vi "Oil Test Sequencer.vi"() -> ()   [LabVIEW 2015]
uses:
  User Interface/Controls/Abort Test.ctl
  User Interface/Controls/Start Test.ctl
  User Interface/Controls/Configuration.ctl
  User Interface/Controls/Manual.ctl
  User Interface/Controls/Quit.ctl
  User Interface/UI Handler/Typedefs/Session Handle.ctl
  User Interface/UI Handler/UI Handler.lvclass
  Tests/Controls/Test Results.ctl
  Tests/Controls/Step Result.ctl
  Tests/Controls/Startup Test.ctl
  Common/Circular Error Log/Typedefs/Session Handle.ctl
  Common/Circular Error Log/Circular Error Log.lvclass
  Tests/Controls/Test Information.ctl
  Tests/Controls/Vacuum Test.ctl
  Tests/Controls/Test Timing.ctl
  Tests/Controls/Vaccum Thresholds.ctl
  Tests/Controls/Helium Test.ctl
  Tests/Controls/Helium Thresholds.ctl
  Tests/Controls/Startup Thresholds.ctl
  User Interface/UI Handler/Typedefs/References.ctl
  Report/Controls/Report Config.ctl
  Common/State Machine/State Machine.lvlib
  Common/Buffers/Snapshot/Snapshot.lvclass
  CAN Communication/Oil/Oil.lvclass
panel:
  in  "Quit":T1
  in  "Manual":T2
  in  "Configuration":T3
  in  "Start Test":T4
  in  "Abort Test":T5
  in  "Configuration Files Path":path=path "C:/TMxFlexTests/OC Assembly Tests/Configuration/ProductionTestConfig.xml"
  in  "User":string
  in  "Serial Number":string="OCxxxxxx"
  in  "Test":string
  out "Time Remaining (s)":dbl
  out "Current Step":dbl
  out "Leak Rate":dbl caption="Leak Rate (PSI/s)" format="%.3f"
  out "NI-DAQ":dbl caption="Test Pressure (PSI)" format="%.3f"
  out "exit":bool
  in  "Display":string
  in  "Test Sequence":i32(listbox)=-2
  in  "Message Log":string
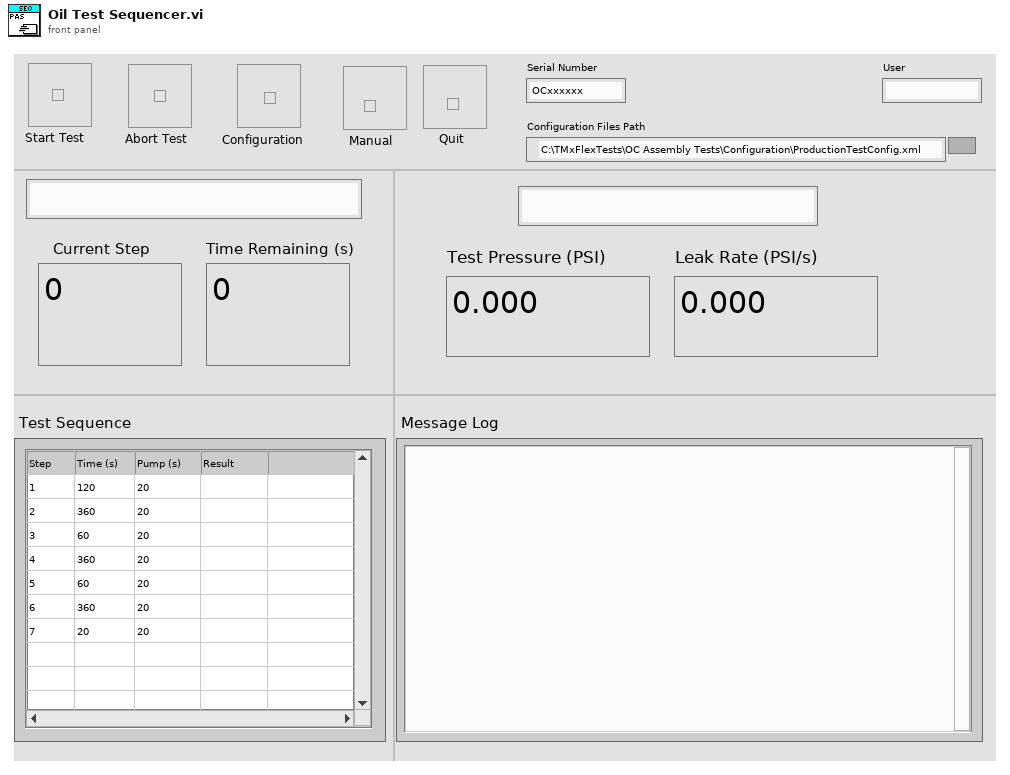
[diagram p1: front panel]
types:
  T1 = typedef "Quit.ctl" = bool
  T2 = typedef "Manual.ctl" = bool
  T3 = typedef "Configuration.ctl" = bool
  T4 = typedef "Start Test.ctl" = bool
  T5 = typedef "Abort Test.ctl" = bool
  T6 = enum8{"Enabled", "Disabled", "Disabled and Grayed Out"}
  T7 = typedef "UI Handler.lvclass/Session Handle.ctl" = refnum<data-value>
  T8 = typedef "Test Results.ctl" = cluster{"Vacuum Test":T9[], "Helium Test":T9[], "Aborted?":bool, "Reason":string, "Abort Time":timestamp, "Test Start":timestamp, "Test End":timestamp, "Startup Test":T10}
  T9 = typedef "Step Result.ctl" = cluster{"Functional Pressure":dbl, "Leak Pressure":dbl, "Func Pass?":bool, "Leak Pass?":bool, "Step Start":timestamp, "Step End":timestamp}
  T10 = typedef "Startup Test.ctl" = cluster{"MIO":dbl, "Temperature":dbl, "MIO Pass?":bool, "Temperature Pass?":bool, "Startup Test Pass?":bool, "Startup Test Start":timestamp, "Startup Test End":timestamp, "Pressure Pass?":bool, "Pressure":dbl}
  T11 = typedef "Circular Error Log.lvclass/Session Handle.ctl" = refnum<data-value>
  T12 = typedef "Test Information.ctl" = cluster{"Vacuum Test":T13, "Helium Test":T16, "Startup Thresholds":T18}
  T13 = typedef "Vacuum Test.ctl" = cluster{"Vacuum Timings":T14[], "Vacuum Thresholds":T15[], "Leak Reasons":string[], "Func Reasons":string[], "FuncSpecEqual":string[], "LeakSpecEqual":string[]}
  T14 = typedef "Test Timing.ctl" = cluster{"Step Wait":dbl, "Pump Wait":dbl}
  T15 = typedef "Vaccum Thresholds.ctl" = cluster{"Func Max Pressure":dbl, "Func Min Pressure":dbl, "Leak Max Pressure":dbl, "Leak Min Pressure":dbl}
  T16 = typedef "Helium Test.ctl" = cluster{"Helium Timings":T14[], "Helium Thresholds":T17[], "Failure Reasons":string[], "LeakSpecEqual":string[]}
  T17 = typedef "Helium Thresholds.ctl" = cluster{"Leak Max Pressure":dbl, "Leak Min Pressure":dbl}
  T18 = typedef "Startup Thresholds.ctl" = cluster{"MIO Max":dbl, "MIO Min":dbl, "Temp Max":dbl, "Temp Min":dbl, "Pressure Max":dbl, "Pressure Min":dbl}
  T19 = cluster{"State":refnum<queue>, "UI Handler":T7, "Serial Number":string, "Test Type":string, "Test Results":T8, "Error":T11, "Operator":string, "config path":path, "Test Configuration":T12}
  T20 = typedef "UI Handler.lvclass/References.ctl" = cluster{"Step":refnum<vi>, "Time":refnum<vi>, "Sequencer":refnum<vi>, "Log":refnum<vi>}
  T21 = cluster{"Serial Number Out":string, "Operator":string}
  T22 = typedef "Report Config.ctl" = cluster{"Serial Number":string, "Test Results":T8, "Operator":string, "Config Filepath":path, "Test Information":T12}
  T23 = typedef "Oil.lvclass/Session Handle.ctl" = refnum<data-value>
  T24 = typedef "Snapshot.lvclass/Session Handle.ctl" = refnum<data-value>
  T25 = typedef "User Configuration.ctl" = cluster{"Password":string, "cDAQ Name":string, "CAN Interface":string}
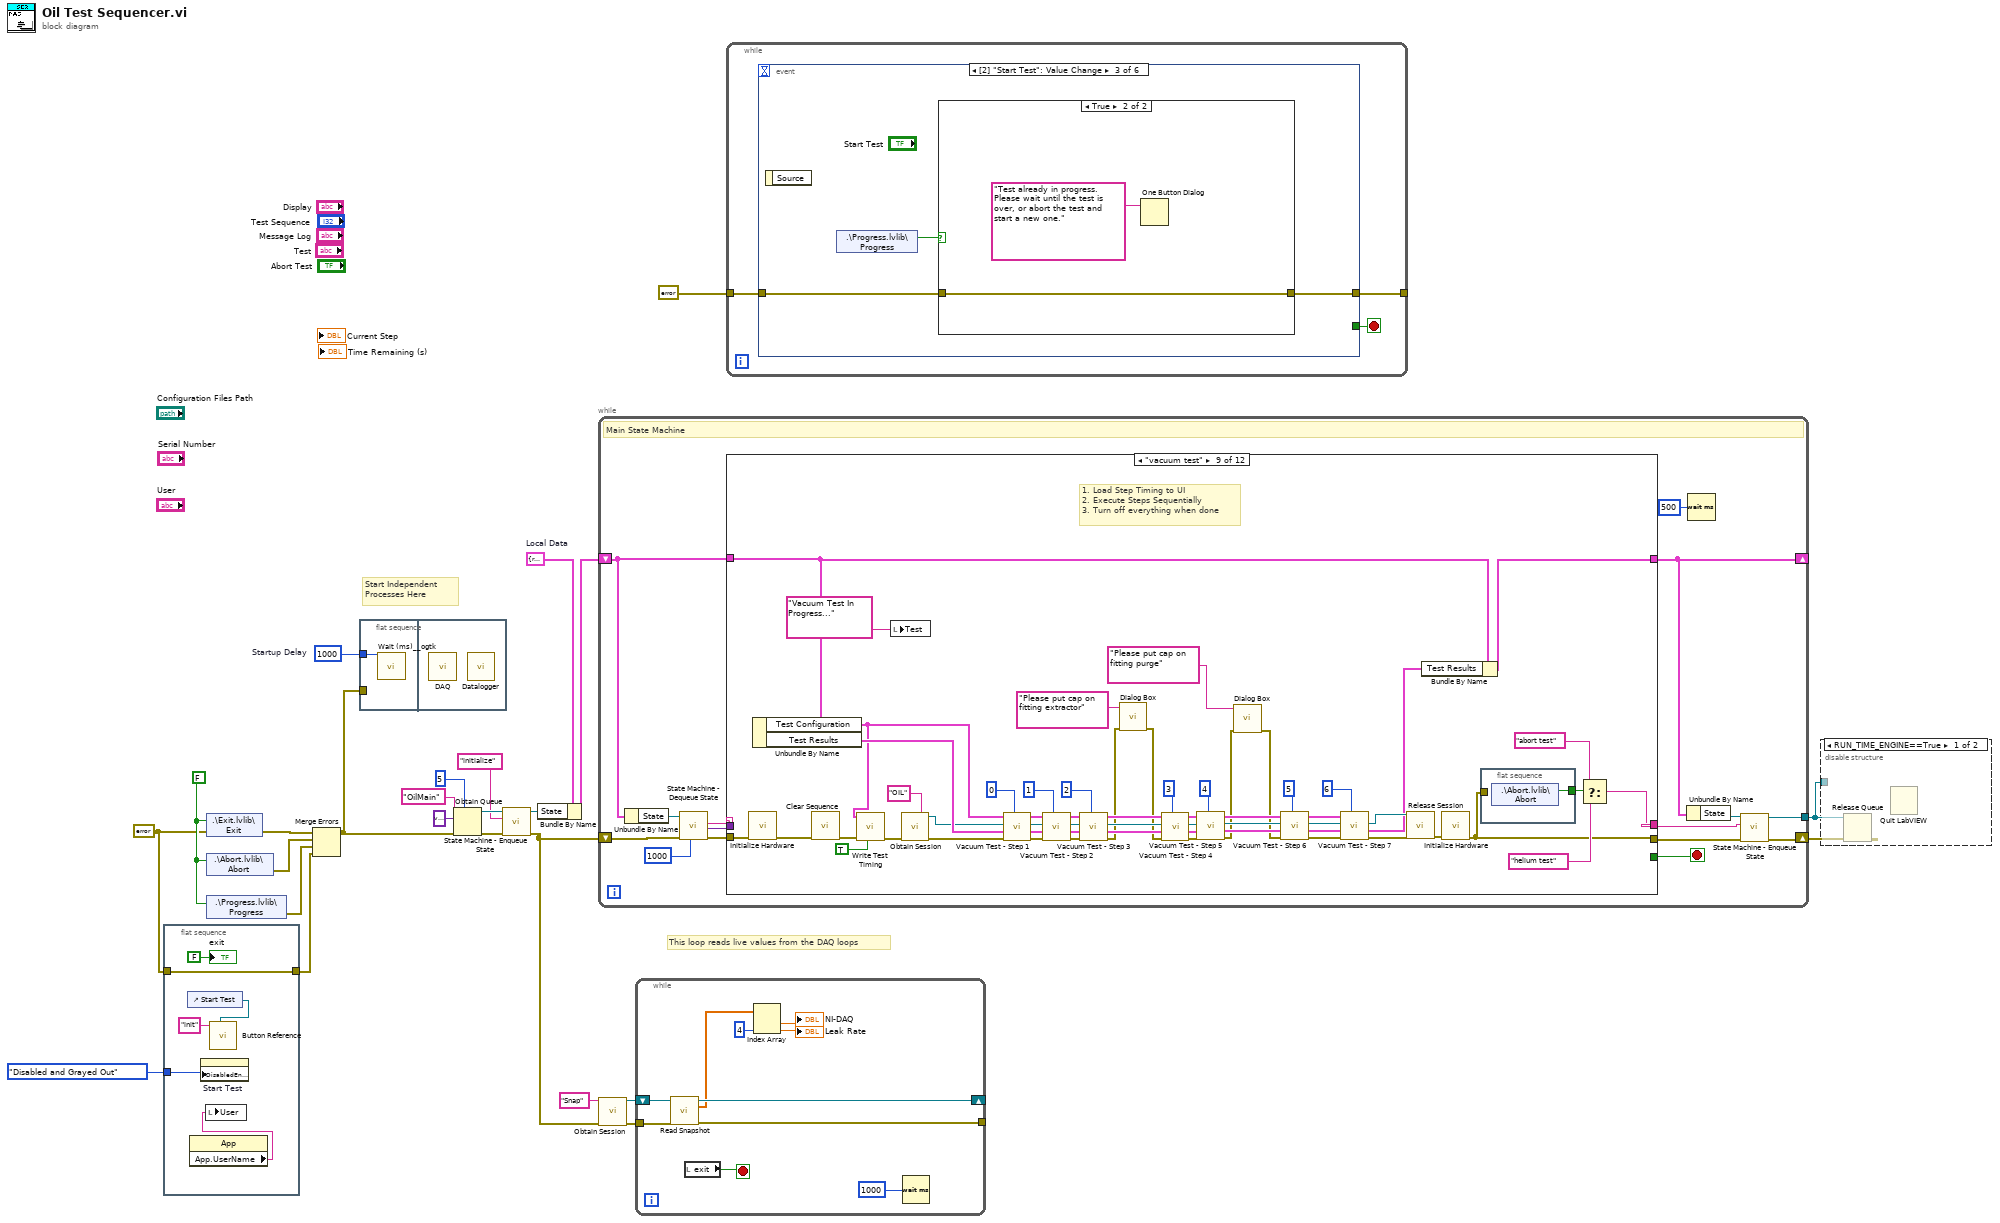
[diagram p0: block diagram]
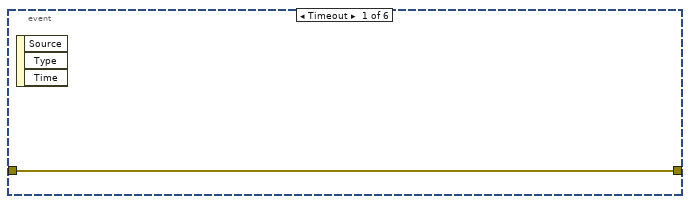
[diagram p3: hidden frame]
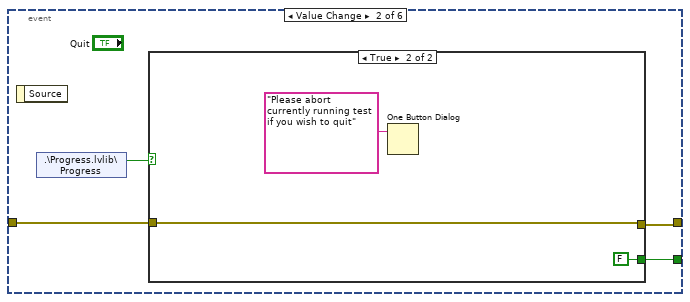
[diagram p4: hidden frame]
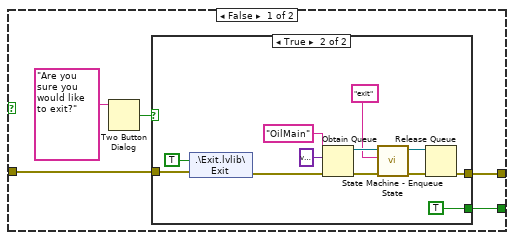
[diagram p5: hidden frame]
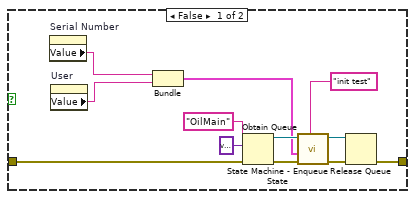
[diagram p7: hidden frame]
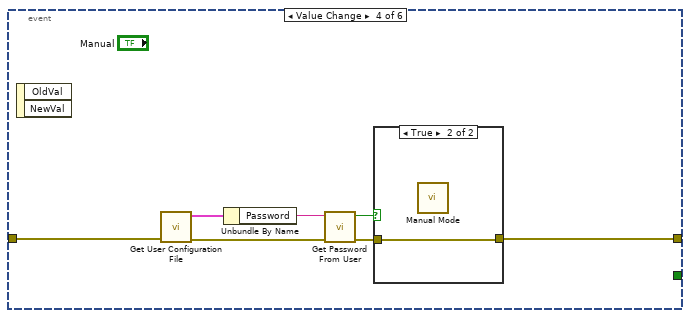
[diagram p8: hidden frame]
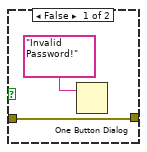
[diagram p9: hidden frame]
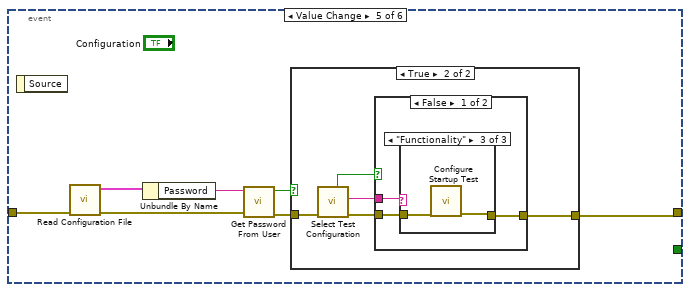
[diagram p10: hidden frame]
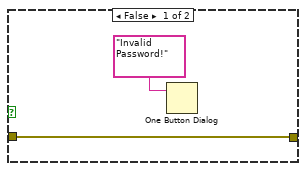
[diagram p11: hidden frame]
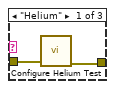
[diagram p12: hidden frame]
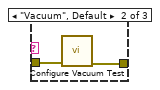
[diagram p13: hidden frame]
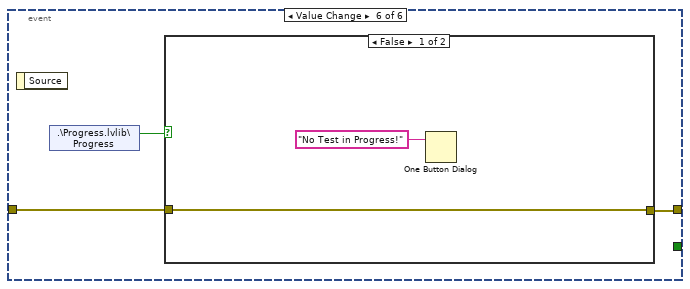
[diagram p15: hidden frame]
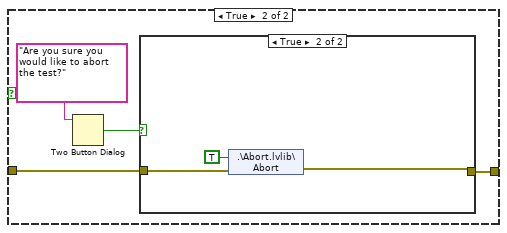
[diagram p16: hidden frame]
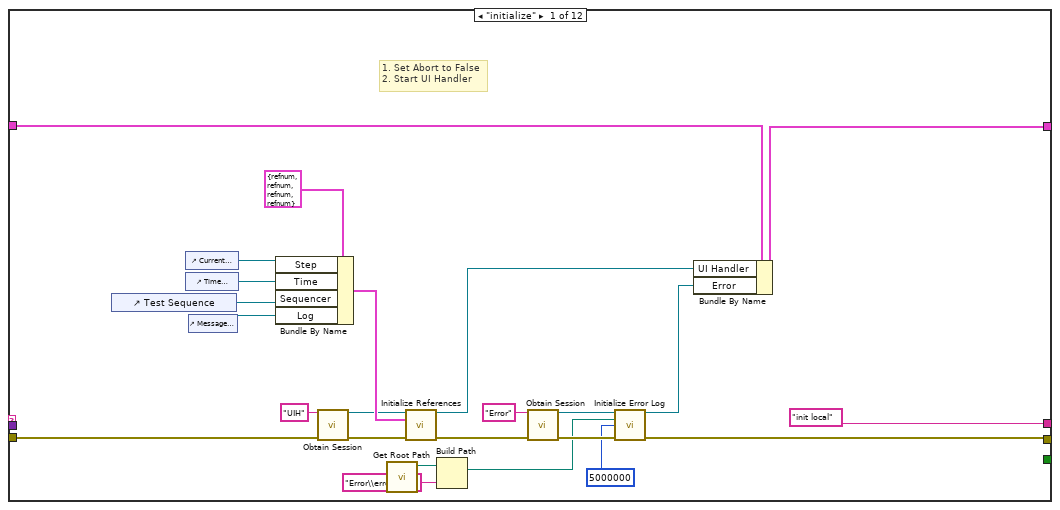
[diagram p18: hidden frame]
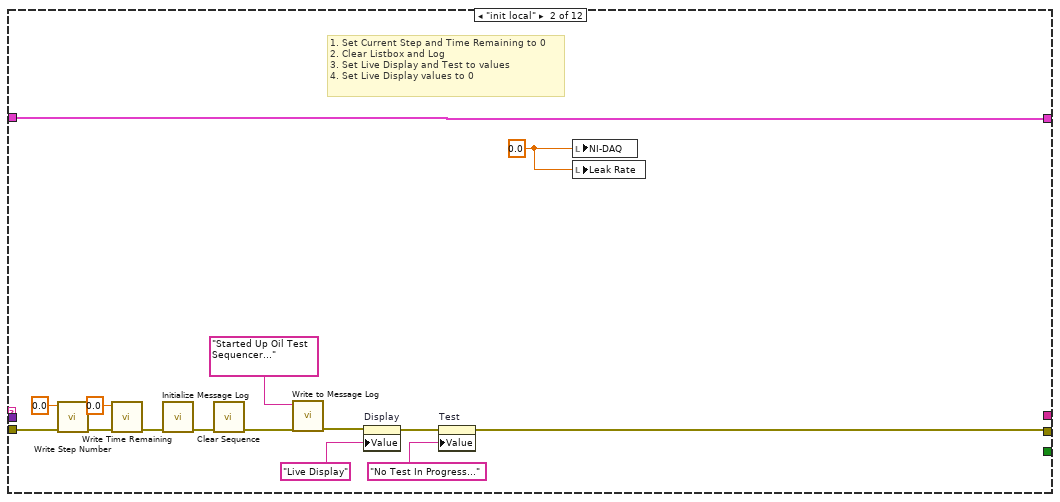
[diagram p19: hidden frame]
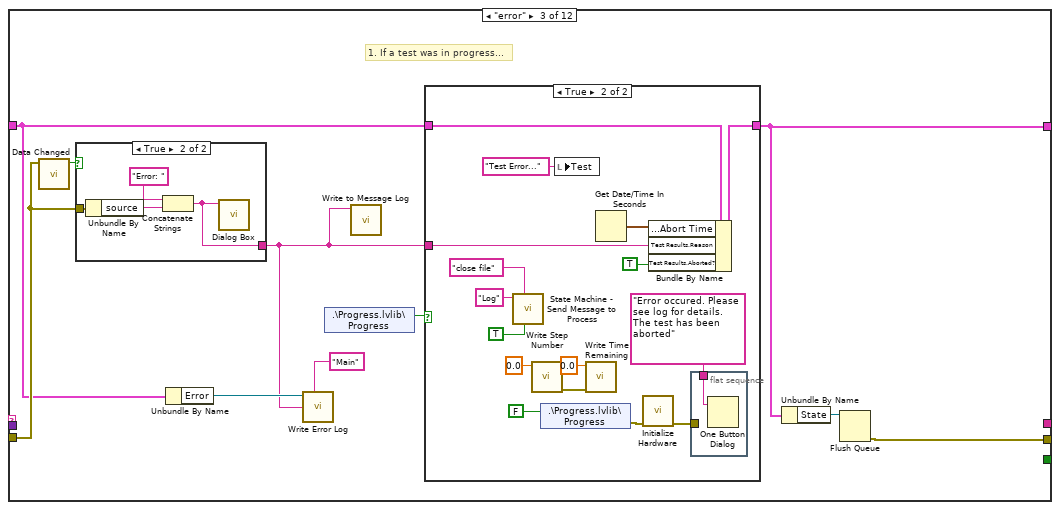
[diagram p20: hidden frame]
diagram:
  w10 = FALSE ("Exit")
  w16 = u32 1000  # Startup Delay
  w4 = errorcluster {"status"=FALSE, "code"=0, "source"=""} ("error in (no error)")
  w19 = T19 {"State"=refnum, "UI Handler"=refnum, "Serial Number"="", "Test Type"="", "Test Results"={"Vacuum Test"=[], "Helium Test"=[], "Aborted?"=FALSE, "Reason"="", "Abort Time"=timestamp(0 s since 1904-01-01), "Test Start"=timestamp(0 s since 1904-01-01), "Test End"=timestamp(0 s since 1904-01-01), "Startup Test"={"MIO"=0.0, "Temperature"=0.0, "MIO Pass?"=FALSE, "Temperature Pass?"=FALSE, "Startup Test Pass?"=FALSE, "Startup Test Start"=timestamp(0 s since 1904-01-01), "Startup Test End"=timestamp(0 s since 1904-01-01), "Pressure Pass?"=FALSE, "Pressure"=0.0}}, "Error"=refnum, "Operator"="", "config path"=path "", "Test Configuration"={"Vacuum Test"={"Vacuum Timings"=[], "Vacuum Thresholds"=[], "Leak Reasons"=[], "Func Reasons"=[], "FuncSpecEqual"=[], "LeakSpecEqual"=[]}, "Helium Test"={"Helium Timings"=[], "Helium Thresholds"=[], "Failure Reasons"=[], "LeakSpecEqual"=[]}, "Startup Thresholds"={"MIO Max"=0.0, "MIO Min"=0.0, "Temp Max"=0.0, "Temp Min"=0.0, "Pressure Max"=0.0, "Pressure Min"=0.0}}}  # Local Data
  # "This loop reads live values from the DAQ loops"
  # "Start Independent\nProcesses Here"
  n1 = flat-sequence {
    tunnel: w4 -> [w30]
    tunnel: [w30] -> w3
    tunnel: T6."Disabled and Grayed Out" ("Disabled") -> [w28]
    frame #0 {
      n2 = control-ref of="Start Test"() -> (w29:refnum<vi>)
      n3 = property class="App"() -> ("App.UserName"=w26:string)  [unwired: 2 in, 2 out]
      n4 = property on="Start Test" class="Bool"("DisabledEnum"=w28) -> ()  [unwired: 2 in, 2 out]
      n5 = local write "User"(w26) -> ()
      n6 = call "Button Reference.vi"("Ref In"=w29, "Command"="init") -> ()  [unwired: 9 in, 1 out]
      "exit" <- FALSE ("exit")
    }
  }
  n7 = shared-variable ".\\Exit.lvlib\\Exit"(w10, error in=w4) -> (error out=w14:errorcluster)
  n8 = shared-variable ".\\Abort.lvlib\\Abort"(w10) -> (error out=w15:errorcluster)  [unwired: 1 in]
  n9 = shared-variable ".\\Progress.lvlib\\Progress"(w10) -> (error out=w9:errorcluster)  [unwired: 1 in]
  n10 = Merge Errors(w14, w15, w9, w3) -> (w13:errorcluster)
  n11 = flat-sequence {
    tunnel: w13 -> [_]
    tunnel: w16 -> [w32]
    frame #0 {
      n12 = call <userlib>:"Wait (ms)__ogtk.vi"("milliseconds to wait"=w32) -> ()  [unwired: 9 in, 2 out]
    }
    frame #1 {
      n13 = call "DAQ.vi"() -> ()  [unwired: 12 in]
      n14 = call "Datalogger.vi"() -> ()  [unwired: 12 in]
    }
  }
  n15 = Obtain Queue(max queue size (-1, unlimited)=5, name (unnamed)="OilMain", element data type=variant, error in (no error)=w13) -> (queue out=w21:refnum<queue>, error out=w22:errorcluster)  [unwired: 1 in, 1 out]
  n16 = call "State Machine - Enqueue State.vi"("error in (no error)"=w22, "State"="initialize", "Queue In"=w21) -> ("error out"=w7:errorcluster, "Queue Out"=w18:refnum<queue>)  [unwired: 7 in]
  n17 = Bundle By Name(cluster=w19, "State"=w18) -> (w17:T19)
  n18 = while "Main State Machine" {
    shift-right: [w44] -> w11
    shift-left: w7 -> [w47]
    shift-right: [w35] -> _
    shift-left: w17 -> [w38]
    tunnel: [w33] -> w2
    stop <- w40 stop-if-true
    # "Main State Machine"
    n19 = Unbundle By Name(w38) -> ("State"=w37:refnum<queue>)
    n20 = call "State Machine - Dequeue State.vi"("Timeout"=1000, "error in (no error)"=w47, "Queue In"=w37) -> ("error out"=w46:errorcluster, "Data"=w34:variant, "State"=w45:string)  [unwired: 4 in, 2 out]
    n21 = case shown="\"vacuum test\"" w45 {
      tunnel: w46 -> [w61 w85 w90 w124 w126 w133 w175 w185 w236 w274 w314 w326]
      tunnel: [w52 w73 w96 w124 w126 w134 w153 w176 w235 w277 w290 w324] -> w43
      tunnel: ["init local" ("State") _ _ _ _ _ w169 "vacuum test" ("Next Test") w237 w278 _ _] -> w42
      tunnel: [_ _ _ _ _ TRUE _ _ _ _ _ _] -> w40
      tunnel: w38 -> [w60 w86 w89 w123 w125 w140 w172 w182 w242 w283 w310 w323]
      tunnel: [w59 w86 w94 w123 w125 w140 w173 w184 w241 w282 w310 w323] -> w35
      tunnel: w34 -> [_ _ _ _ _ _ w174 _ _ _ _ _]
      frame "initialize" {
        # "1. Set Abort to False\n2. Start UI Handler"
        n22 = control-ref of="Test Sequence"() -> (w64:refnum<vi>)
        n23 = control-ref of="Current Step"() -> (w62:refnum<vi>)
        n24 = control-ref of="Time Remaining (s)"() -> (w63:refnum<vi>)
        n25 = control-ref of="Message Log"() -> (w65:refnum<vi>)
        n26 = Bundle By Name(cluster=T20 {"Step"=refnum, "Time"=refnum, "Sequencer"=refnum, "Log"=refnum} ("References"), "Step"=w62, "Time"=w63, "Sequencer"=w64, "Log"=w65) -> (w70:T20)
        n27 = call "Obtain Session.vi"("Session  Name ()"="UIH", "error in (no error)"=w61) -> ("Session Handle"=w68:T7, "error out"=w69:errorcluster)  [unwired: 12 in]
        n28 = call "Get Root Path.vi"() -> ("Root Path"=w50:path)  [unwired: 11 in]
        n29 = call "Initialize References.vi"("Session Handle in"=w68, "References"=w70, "error in (no error)"=w69) -> ("Session Handle out"=w58:T7, "error out"=w57:errorcluster)  [unwired: 11 in]
        n30 = Build Path(base path=w50, name or relative path="Error\\error.txt") -> (appended path=w48:path)
        n31 = call "Obtain Session.vi"("Session  Name ()"="Error", "error in (no error)"=w57) -> ("Session Handle"=w54:T11, "error out"=w55:errorcluster)  [unwired: 12 in]
        n32 = call "Initialize Error Log.vi"("Session Handle in"=w54, "Error Path"=w48, "Max File Size"=i64 5000000, "error in (no error)"=w55) -> ("Session Handle out"=w51:T11, "error out"=w52:errorcluster)  [unwired: 10 in]
        n33 = Bundle By Name(cluster=w60, "UI Handler"=w58, "Error"=w51) -> (w59:T19)
      }
      frame "init local" {
        w72 = 0.0 ("Test Pressure (PSI)")
        # "1. Set Current Step and Time Remaining to 0\n2. Clear Listbox and Log\n3. Set Live Display and Test to values \n4. Set Live Display values to 0"
        n34 = call "Write Step Number.vi"("error in (no error)"=w85, "Value"=0.0) -> ("error out"=w83:errorcluster)  [unwired: 9 in]
        n35 = call "Write Time Remaining.vi"("error in (no error)"=w83, "Value"=0.0) -> ("error out"=w81:errorcluster)  [unwired: 9 in]
        n36 = call "Initialize Message Log.vi"("error in (no error)"=w81) -> ("error out"=w80:errorcluster)  [unwired: 10 in]
        n37 = call "Clear Sequence.vi"("error in (no error)"=w80) -> ("error out"=w79:errorcluster)  [unwired: 10 in]
        n38 = call "Write to Message Log.vi"("error in (no error)"=w79, "Message"="Started Up Oil Test Sequencer...") -> ("error out"=w77:errorcluster)  [unwired: 9 in]
        n39 = property on="Display" class="Str"(error in=w77, "Value"="Live Display" ("Display")) -> (error out=w75:errorcluster)  [unwired: 1 in, 1 out]
        n40 = property on="Test" class="Str"(error in=w75, "Value"="No Test In Progress..." ("Test")) -> (error out=w73:errorcluster)  [unwired: 1 in, 1 out]
        n41 = local write "NI-DAQ"(w72) -> ()
        n42 = local write "Leak Rate"(w72) -> ()
      }
      frame "error" {
        # "1. If a test was in progress..."
        n43 = call "Data Changed.vi"("Data"=w90) -> ("Changed?"=w92:bool)  [unwired: 10 in]
        n44 = case shown="True" w92 {
          tunnel: [w97 w101] -> w87
          tunnel: w90 -> [w98 w102]
          frame False {
            n45 = Unbundle By Name(w98) -> ("source"=w99:string)
            n46 = Concatenate Strings("Error: " ("string"), w99) -> (w97:string)
          }
          frame True {
            n47 = Unbundle By Name(w102) -> ("source"=w103:string)
            n48 = Concatenate Strings("Error: " ("string"), w103) -> (w101:string)
            n49 = call "Dialog Box.vi"("Serial Number"=w101) -> ()  [unwired: 10 in, 1 out]
          }
        }
        n50 = Unbundle By Name(w89) -> ("Error"=w88:T11)
        n51 = call "Write Error Log.vi"("Session Handle in"=w88, "Process Name"="Main", "Data"=w87) -> ()  [unwired: 11 in, 2 out]
        n52 = shared-variable ".\\Progress.lvlib\\Progress"() -> (w93:bool)  [unwired: 1 in, 1 out]
        n53 = call "Write to Message Log.vi"("Message"=w87) -> ()  [unwired: 10 in, 1 out]
        n54 = case shown="True" w93 {
          tunnel: w89 -> [w105 w120]
          tunnel: [w105 w119] -> w94
          tunnel: w87 -> [_ w117]
          frame False {
          }
          frame True {
            n55 = call "State Machine - Send Message to Process.vi"("Front?"=TRUE, "State"="close file", "Process Name"="Log") -> ()  [unwired: 8 in, 1 out]
            n56 = call "Write Step Number.vi"("Value"=0.0) -> ("error out"=w110:errorcluster)  [unwired: 10 in]
            n57 = shared-variable ".\\Progress.lvlib\\Progress"(FALSE ("Progress")) -> (error out=w115:errorcluster)  [unwired: 1 in]
            n58 = local write "Test"("Test Error..." ("Test")) -> ()
            n59 = call "Write Time Remaining.vi"("error in (no error)"=w110, "Value"=0.0) -> ()  [unwired: 9 in, 1 out]
            n60 = Get Date/Time In Seconds() -> (seconds since 1Jan1904=w118:timestamp)
            n61 = call "Initialize Hardware.vi"("error in"=w115) -> ("error out"=w114:errorcluster)  [unwired: 10 in]
            n62 = Bundle By Name(cluster=w120, "Test Results.Abort Time"=w118, "Test Results.Reason"=w117, "Test Results.Aborted?"=TRUE) -> (w119:T19)
            n63 = flat-sequence {
              tunnel: w114 -> [_]
              tunnel: "Error occured. Please see log for details. The test has been aborted" -> [w122]
              frame #0 {
                n64 = One Button Dialog(message=w122) -> ()  [unwired: 1 in, 1 out]
              }
            }
          }
        }
        n65 = Unbundle By Name(w94) -> ("State"=w95:refnum<queue>)
        n66 = Flush Queue(queue=w95) -> (error out=w96:errorcluster)  [unwired: 1 in, 2 out]
      }
      frame Default {
      }
      frame "idle" {
      }
      frame "exit" {
        # "1. Clean up all references\n2. Exit commands to Datalogger"
        n67 = Unbundle By Name(w140) -> ("UI Handler"=w139:T7)
        n68 = call "Write to Message Log.vi"("error in (no error)"=w133, "Message"="Initializing Hardware before exit") -> ("error out"=w132:errorcluster)  [unwired: 9 in]
        n69 = call "Initialize Hardware.vi"("error in"=w132) -> ("error out"=w130:errorcluster)  [unwired: 10 in]
        n70 = call "Release Session.vi"("Session Handle"=w139, "error in (no error)"=w130) -> ()  [unwired: 13 in, 1 out]
        n71 = local write "exit"(TRUE ("exit")) -> ()
        n72 = call "State Machine - Send Message to Process.vi"("Front?"=TRUE, "State"="exit", "Process Name"="DAQ") -> ("error out"=w134:errorcluster)  [unwired: 8 in]
        n73 = call "State Machine - Send Message to Process.vi"("Front?"=TRUE, "State"="exit", "Process Name"="Log") -> ()  [unwired: 8 in, 1 out]
      }
      frame "init test" {
        # "Read test config"
        # "1. Initialize all Hardware\n2. Store Serial Number\n3. Send start command to logger\n4.. Proceed to Test"
        n74 = Variant To Data(error in=w175, type=T21 {"Serial Number Out"="", "Operator"=""} ("cluster"), Variant=w174) -> (data=w168:T21, error out=w145:errorcluster)
        n75 = property on="Configuration Files Path" class="Path"() -> ("Value"=w142:path)  [unwired: 2 in, 2 out]
        n76 = call "Read Test Information From File.vi"("error in"=w145, "file (use dialog)"=w142) -> ("error out"=w144:errorcluster, "Test Information"=w143:T12)  [unwired: 8 in]
        n77 = call "Obtain Session.vi"("Session  Name ()"="OIL", "error in (no error)"=w144) -> ("Session Handle"=w162:T23, "error out"=w163:errorcluster)  [unwired: 12 in]
        n78 = call "Get Device Status.vi"("Session Handle in"=w162, "error in (no error)"=w163) -> ("Session Handle out"=w159:T23, "error out"=w161:errorcluster)  [unwired: 11 in, 1 out]
        n79 = Unbundle By Name(w168) -> ("Operator"=w165:string, "Serial Number Out"=w147:string)
        n80 = call "Write to Message Log.vi"("error in (no error)"=w161, "Message"="Initializing Hardware...") -> ("error out"=w158:errorcluster)  [unwired: 9 in]
        n81 = call "Initialize Hardware.vi"("error in"=w158) -> ("error out"=w148:errorcluster)  [unwired: 10 in]
        n82 = call "WriteVerify Mfg Serial Number.vi"("error in"=w148, "Serial Number"=w147) -> ("error out"=w146:errorcluster)  [unwired: 9 in]
        n83 = Bundle("Serial Number Out"=w147) -> (w149:cluster{"Serial Number Out":string})  [unwired: 1 in]
        n84 = call "State Machine - Send Message to Process.vi"("Data"=w149, "Front?"=TRUE, "State"="create path", "Process Name"="Log") -> ()  [unwired: 7 in, 1 out]
        n85 = call "Release Session.vi"("Session Handle"=w159, "error in (no error)"=w146) -> ("error out"=w156:errorcluster)  [unwired: 13 in]
        n86 = call "Dialog Box.vi"("error in (no error)"=w156, "Serial Number"="Please ensure that there is a cap on the CHV 1 PSI Fitting. Extractor and purge fittings should not be capped.") -> ("error out"=w154:errorcluster)  [unwired: 9 in]
        n87 = Bundle By Name(cluster=w172, "Test Results"=T8 {"Vacuum Test"=[], "Helium Test"=[], "Aborted?"=FALSE, "Reason"="", "Abort Time"=timestamp(0 s since 1904-01-01), "Test Start"=timestamp(0 s since 1904-01-01), "Test End"=timestamp(0 s since 1904-01-01), "Startup Test"={"MIO"=0.0, "Temperature"=0.0, "MIO Pass?"=FALSE, "Temperature Pass?"=FALSE, "Startup Test Pass?"=FALSE, "Startup Test Start"=timestamp(0 s since 1904-01-01), "Startup Test End"=timestamp(0 s since 1904-01-01), "Pressure Pass?"=FALSE, "Pressure"=0.0}}, "Operator"=w165, "Serial Number"=w147, "config path"=w142, "Test Configuration"=w143) -> (w173:T19)
        n88 = call "Clear Sequence.vi"("error in (no error)"=w154) -> ("error out"=w153:errorcluster)  [unwired: 10 in]
        n89 = Select(t="startup test" ("Error String"), s=TRUE ("Progress"), f="idle" ("Error String")) -> (s? t:f=w169:string)
      }
      frame "startup test" {
        # "1. Oil Pump Test\n2. MIO , Temp, Pressure readings"
        n90 = shared-variable ".\\Progress.lvlib\\Progress"(TRUE ("Progress"), error in=w185) -> (error out=w180:errorcluster)
        n91 = Unbundle By Name(w182) -> ("Test Configuration"=w181:T12, "Test Results"=w179:T8)
        n92 = local write "Test"("Startup Test in Progress..." ("Test")) -> ()
        n93 = call "Startup Test.vi"("error in"=w180, "Test Results In"=w179, "Test Configuration In"=w181) -> ("error out"=w176:errorcluster, "Test Results Out"=w178:T8)  [unwired: 6 in, 1 out]
        n94 = Bundle By Name(cluster=w182, "Test Results"=w178) -> (w184:T19)
      }
      frame "vacuum test" {
        # "1. Load Step Timing to UI\n2. Execute Steps Sequentially\n3. Turn off everything when done"
        n95 = call "Initialize Hardware.vi"("error in"=w236) -> ("error out"=w233:errorcluster)  [unwired: 10 in]
        n96 = Unbundle By Name(w242) -> ("Test Configuration"=w207:T12, "Test Results"=w234:T8)
        n97 = call "Clear Sequence.vi"("error in (no error)"=w233) -> ("error out"=w232:errorcluster)  [unwired: 10 in]
        n98 = call "Write Test Timing.vi"("Vacuum?"=TRUE, "error in (no error)"=w232, "Test Configuration"=w207) -> ("error out"=w228:errorcluster)  [unwired: 8 in]
        n99 = local write "Test"("Vacuum Test In Progress..." ("Test")) -> ()
        n100 = call "Obtain Session.vi"("Session  Name ()"="OIL", "error in (no error)"=w228) -> ("Session Handle"=w195:T23, "error out"=w196:errorcluster)  [unwired: 12 in]
        n101 = call "Vacuum Test - Step 1.vi"("Step"=0, "error in"=w196, "Test Results"=w234, "Oil In"=w195, "Test Configuration"=w207) -> ("error out"=w226:errorcluster, "Test Results Out"=w225:T8, "Oil Out"=w224:T23, "Test Configuration Out"=w223:T12)  [unwired: 3 in]
        n102 = call "Vacuum Test - Step 2.vi"("Step"=1, "error in"=w226, "Test Results"=w225, "Oil In"=w224, "Test Configuration"=w223) -> ("error out"=w221:errorcluster, "Test Results Out"=w220:T8, "Oil Out"=w219:T23, "Test Configuration Out"=w218:T12)  [unwired: 3 in]
        n103 = call "Vacuum Test - Step 3.vi"("Step"=2, "error in"=w221, "Test Results"=w220, "Oil In"=w219, "Test Configuration"=w218) -> ("error out"=w201:errorcluster, "Test Results Out"=w216:T8, "Oil Out"=w215:T23, "Test Configuration Out"=w214:T12)  [unwired: 3 in]
        n104 = call "Dialog Box.vi"("error in (no error)"=w201, "Serial Number"="Please put cap on fitting extractor") -> ("error out"=w200:errorcluster)  [unwired: 9 in]
        n105 = call "Vacuum Test - Step 4.vi"("Step"=3, "error in"=w200, "Test Results"=w216, "Oil In"=w215, "Test Configuration"=w214) -> ("error out"=w212:errorcluster, "Test Results Out"=w211:T8, "Oil Out"=w210:T23, "Test Configuration Out"=w209:T12)  [unwired: 3 in]
        n106 = call "Vacuum Test - Step 5.vi"("Step"=4, "error in"=w212, "Test Results"=w211, "Oil In"=w210, "Test Configuration"=w209) -> ("error out"=w199:errorcluster, "Test Results Out"=w204:T8, "Oil Out"=w205:T23, "Test Configuration Out"=w206:T12)  [unwired: 3 in]
        n107 = call "Dialog Box.vi"("error in (no error)"=w199, "Serial Number"="Please put cap on fitting purge") -> ("error out"=w198:errorcluster)  [unwired: 9 in]
        n108 = call "Vacuum Test - Step 6.vi"("Step"=5, "error in"=w198, "Test Results"=w204, "Oil In"=w205, "Test Configuration"=w206) -> ("error out"=w189:errorcluster, "Test Results Out"=w191:T8, "Oil Out"=w194:T23, "Test Configuration Out"=w192:T12)  [unwired: 3 in]
        n109 = call "Vacuum Test - Step 7.vi"("Step"=6, "error in"=w189, "Test Results"=w191, "Oil In"=w194, "Test Configuration"=w192) -> ("error out"=w188:errorcluster, "Test Results Out"=w190:T8, "Oil Out"=w193:T23)  [unwired: 3 in, 1 out]
        n110 = call "Release Session.vi"("Session Handle"=w193, "error in (no error)"=w188) -> ("error out"=w227:errorcluster)  [unwired: 13 in]
        n111 = Bundle By Name(cluster=w242, "Test Results"=w190) -> (w241:T19)
        n112 = call "Initialize Hardware.vi"("error in"=w227) -> ("error out"=w235:errorcluster)  [unwired: 10 in]
        n113 = flat-sequence {
          tunnel: [w244] -> w240
          tunnel: w235 -> [_]
          frame #0 {
            n114 = shared-variable ".\\Abort.lvlib\\Abort"() -> (w244:bool)  [unwired: 1 in, 1 out]
          }
        }
        n115 = Select(t="abort test" ("Next Test"), s=w240, f="helium test" ("Next Test")) -> (s? t:f=w237:string)
      }
      frame "helium test" {
        # "1. Load Step Timing to UI\n2. Execute Steps Sequentially\n3. Turn off everything when done"
        n116 = Unbundle By Name(w283) -> ("Test Configuration"=w264:T12, "Test Results"=w276:T8)
        n117 = case shown="No Error" w274 {
          selector: w274 -> [w287 w288]
          tunnel: [w286 w288] -> w273
          tunnel: "Press OK to continue to Helium Test..." ("Test") -> [w285 _]
          frame No Error {
            n118 = call "Dialog Box.vi"("error in (no error)"=w287, "Serial Number"=w285) -> ("error out"=w286:errorcluster)  [unwired: 9 in]
          }
          frame Error {
          }
        }
        n119 = call "Initialize Hardware.vi"("error in"=w273) -> ("error out"=w269:errorcluster)  [unwired: 10 in]
        n120 = local write "Test"("Helium Test In Progress..." ("Test")) -> ()
        n121 = call "Clear Sequence.vi"("error in (no error)"=w269) -> ("error out"=w271:errorcluster)  [unwired: 10 in]
        n122 = call "Write Test Timing.vi"("Vacuum?"=FALSE, "error in (no error)"=w271, "Test Configuration"=w264) -> ("error out"=w267:errorcluster)  [unwired: 8 in]
        n123 = call "Obtain Session.vi"("Session  Name ()"="OIL", "error in (no error)"=w267) -> ("Session Handle"=w265:T23, "error out"=w266:errorcluster)  [unwired: 12 in]
        n124 = call "Helium Test - Step 1.vi"("Step"=0, "error in"=w266, "Test Results"=w276, "Oil In"=w265, "Test Configuration"=w264) -> ("error out"=w260:errorcluster, "Test Results Out"=w261:T8, "Oil Out"=w262:T23, "Test Configuration Out"=w263:T12)  [unwired: 3 in]
        n125 = call "Helium Test - Step 2.vi"("Step"=1, "error in"=w260, "Test Results"=w261, "Oil In"=w262, "Test Configuration"=w263) -> ("error out"=w258:errorcluster, "Test Results Out"=w257:T8, "Oil Out"=w256:T23, "Test Configuration Out"=w255:T12)  [unwired: 3 in]
        n126 = call "Helium Test - Step 3.vi"("Step"=2, "error in"=w258, "Test Results"=w257, "Oil In"=w256, "Test Configuration"=w255) -> ("error out"=w253:errorcluster, "Test Results Out"=w252:T8, "Oil Out"=w251:T23, "Test Configuration Out"=w250:T12)  [unwired: 3 in]
        n127 = call "Helium Test - Step 4.vi"("Step"=3, "error in"=w253, "Test Results"=w252, "Oil In"=w251, "Test Configuration"=w250) -> ("error out"=w247:errorcluster, "Test Results Out"=w248:T8, "Oil Out"=w246:T23)  [unwired: 3 in, 1 out]
        n128 = call "Release Session.vi"("Session Handle"=w246, "error in (no error)"=w247) -> ("error out"=w245:errorcluster)  [unwired: 13 in]
        n129 = call "Initialize Hardware.vi"("error in"=w245) -> ("error out"=w277:errorcluster)  [unwired: 10 in]
        n130 = flat-sequence {
          tunnel: [w289] -> w281
          tunnel: w277 -> [_]
          frame #0 {
            n131 = shared-variable ".\\Abort.lvlib\\Abort"() -> (w289:bool)  [unwired: 1 in, 1 out]
          }
        }
        n132 = Bundle By Name(cluster=w283, "Test Results"=w248) -> (w282:T19)
        n133 = Select(t="abort test" ("Next Test"), s=w281, f="test done" ("Next Test")) -> (s? t:f=w278:string)
      }
      frame "test done" {
        w300 = "OC" ("Fixture Name")
        # "1. Stop Logging\n2. Initialize all HW\n3. Write Report"
        n134 = call "Write to Message Log.vi"("error in (no error)"=w314, "Message"="Test Completed Sucessfully!") -> ("error out"=w308:errorcluster)  [unwired: 9 in]
        n135 = call "Get Date Timestamp.vi"("error in (no error)"=w308) -> ("error out"=w309:errorcluster)  [unwired: 9 in, 1 out]
        n136 = call "Initialize Hardware.vi"("error in"=w309) -> ("error out"=w313:errorcluster)  [unwired: 10 in]
        n137 = local write "Test"("Test Complete..." ("Test")) -> ()
        n138 = shared-variable ".\\Progress.lvlib\\Progress"(FALSE ("Progress"), error in=w313) -> (error out=w294:errorcluster)
        n139 = Unbundle By Name(w310) -> ("Serial Number"=w307:string, "Test Results"=w299:T8, "Test Configuration"=w298:T12, "Operator"=w305:string, "config path"=w304:path)
        n140 = call "Write Step Number.vi"("error in (no error)"=w294, "Value"=0.0) -> ("error out"=w296:errorcluster)  [unwired: 9 in]
        n141 = call "Write Time Remaining.vi"("error in (no error)"=w296, "Value"=0.0) -> ("error out"=w293:errorcluster)  [unwired: 9 in]
        n142 = Bundle By Name(cluster=T22 {"Serial Number"="", "Test Results"={"Vacuum Test"=[], "Helium Test"=[], "Aborted?"=FALSE, "Reason"="", "Abort Time"=timestamp(0 s since 1904-01-01), "Test Start"=timestamp(0 s since 1904-01-01), "Test End"=timestamp(0 s since 1904-01-01), "Startup Test"={"MIO"=0.0, "Temperature"=0.0, "MIO Pass?"=FALSE, "Temperature Pass?"=FALSE, "Startup Test Pass?"=FALSE, "Startup Test Start"=timestamp(0 s since 1904-01-01), "Startup Test End"=timestamp(0 s since 1904-01-01), "Pressure Pass?"=FALSE, "Pressure"=0.0}}, "Operator"="", "Config Filepath"=path "", "Test Information"={"Vacuum Test"={"Vacuum Timings"=[], "Vacuum Thresholds"=[], "Leak Reasons"=[], "Func Reasons"=[], "FuncSpecEqual"=[], "LeakSpecEqual"=[]}, "Helium Test"={"Helium Timings"=[], "Helium Thresholds"=[], "Failure Reasons"=[], "LeakSpecEqual"=[]}, "Startup Thresholds"={"MIO Max"=0.0, "MIO Min"=0.0, "Temp Max"=0.0, "Temp Min"=0.0, "Pressure Max"=0.0, "Pressure Min"=0.0}}} ("Report Info"), "Serial Number"=w307, "Test Results"=w299, "Test Information"=w298, "Operator"=w305, "Config Filepath"=w304) -> (w303:T22)
        n143 = call "Create Report CSV.vi"("error in (no error)"=w293, "Fixture Name"=w300, "Report Info"=w303) -> ("error out"=w301:errorcluster)  [unwired: 8 in]
        n144 = call "Test Summary Page.vi"("error in (no error)"=w301, "Test Configuration"=w298, "Test Results"=w299, "Type"=w300) -> ("error out"=w291:errorcluster, "Result"=w292:bool)  [unwired: 6 in]
        n145 = case shown="True" w292 {
          tunnel: w291 -> [_ w316]
          tunnel: [_ w315] -> w290
          frame False {
          }
          frame True {
            # "Write Tested Date"
            n146 = call "WriteVerify Mfg Test Timestamp.vi"("error in"=w316) -> ("error out"=w315:errorcluster)  [unwired: 10 in]
          }
        }
      }
      frame "abort test" {
        w329 = FALSE ("Progress")
        # "1. Stop logging and init hardware"
        n147 = call "Write to Message Log.vi"("error in (no error)"=w326, "Message"="Test Aborted..." ("Test")) -> ("error out"=w318:errorcluster)  [unwired: 9 in]
        n148 = call "Write Step Number.vi"("error in (no error)"=w318, "Value"=0.0) -> ("error out"=w320:errorcluster)  [unwired: 9 in]
        n149 = local write "Test"("Test Aborted..." ("Test")) -> ()
        n150 = call "Write Time Remaining.vi"("error in (no error)"=w320, "Value"=0.0) -> ("error out"=w317:errorcluster)  [unwired: 9 in]
        n151 = call "Initialize Hardware.vi"("error in"=w317) -> ("error out"=w332:errorcluster)  [unwired: 10 in]
        n152 = shared-variable ".\\Progress.lvlib\\Progress"(w329, error in=w332) -> (error out=w328:errorcluster)
        n153 = shared-variable ".\\Abort.lvlib\\Abort"(w329) -> (error out=w327:errorcluster)  [unwired: 1 in]
        n154 = Merge Errors(w328, w327) -> (w325:errorcluster)
        n155 = Unbundle By Name(w323) -> ("State"=w322:refnum<queue>)
        n156 = Flush Queue(queue=w322, error in (no error)=w325) -> (error out=w324:errorcluster)  [unwired: 2 out]
      }
    }
    n157 = Unbundle By Name(w35) -> ("State"=w36:refnum<queue>)
    n158 = Wait (ms)(milliseconds to wait=u32 500) -> ()  [unwired: 1 out]
    n159 = call "State Machine - Enqueue State.vi"("error in (no error)"=w43, "State"=w42, "Queue In"=w36) -> ("error out"=w44:errorcluster, "Queue Out"=w33:refnum<queue>)  [unwired: 7 in]
  }
  n160 = call "Obtain Session.vi"("Session  Name ()"="Snap", "error in (no error)"=w7) -> ("Session Handle"=w5:T24, "error out"=w6:errorcluster)  [unwired: 12 in]
  n161 = while {
    tunnel: w6 -> [w341]
    shift-right: [w337] -> _
    shift-left: w5 -> [w340]
    tunnel: [w338] -> _
    stop <- w342 stop-if-true
    n162 = call "Read Snapshot.vi"("Session Handle in"=w340, "error in (no error)"=w341) -> ("Session Handle out"=w337:T24, "Buffer"=w336:dbl[], "error out"=w338:errorcluster)  [unwired: 11 in]
    n163 = local read "exit"() -> (w342:bool)
    n164 = Index Array(array=w336, index #2=4 ("index")) -> (element #1=→"NI-DAQ":dbl, element #2=→"Leak Rate":dbl)  [unwired: 1 in]
    n165 = Wait (ms)(milliseconds to wait=u32 1000) -> ()  [unwired: 1 out]
  }
  n166 = while {
    tunnel: errorcluster {"status"=FALSE, "code"=0, "source"=""} ("error in (no error)") -> [w344]
    tunnel: [w343] -> _
    stop <- w345 stop-if-true
    n167 = event shown="[2] \"Start Test\": Value Change" {
      selector: _ -> [_ _ _ _ _ _]
      dyn-events: _ -> [_ _ _ _ _ _]
      timeout: _ -> [_ _ _ _ _ _]
      tunnel: [_ w348 _ _ _ _] -> w345
      tunnel: w344 -> [w346 w349 w374 w395 w402 w425]
      tunnel: [w346 w350 w373 w391 w405 w424] -> w343
      event Timeout {
        n168 = event-data() -> ()  [unwired: 1 in, 3 out]
      }
      event Value Change {
        n169 = event-data() -> ()  [unwired: 1 in, 1 out]
        n170 = shared-variable ".\\Progress.lvlib\\Progress"() -> (w347:bool)  [unwired: 1 in, 1 out]
        n171 = case shown="True" w347 {
          tunnel: [w355 w370] -> w350
          tunnel: w349 -> [w354 w370]
          tunnel: [w351 FALSE] -> w348
          frame False {
            n172 = Two Button Dialog(message="Are you sure you would like to exit?") -> (T button?=w352:bool)  [unwired: 2 in]
            n173 = case shown="True" w352 {
              tunnel: [w356 w361] -> w355
              tunnel: w354 -> [w356 w360]
              tunnel: [_ TRUE] -> w351
              frame False {
              }
              frame True {
                n174 = shared-variable ".\\Exit.lvlib\\Exit"(TRUE ("Exit"), error in=w360) -> (error out=w359:errorcluster)
                n175 = Obtain Queue(name (unnamed)="OilMain", element data type=variant, error in (no error)=w359) -> (queue out=w365:refnum<queue>, error out=w366:errorcluster)  [unwired: 2 in, 1 out]
                n176 = call "State Machine - Enqueue State.vi"("error in (no error)"=w366, "State"="exit", "Queue In"=w365) -> ("error out"=w363:errorcluster, "Queue Out"=w362:refnum<queue>)  [unwired: 7 in]
                n177 = Release Queue(queue=w362, error in (no error)=w363) -> (error out=w361:errorcluster)  [unwired: 1 in, 2 out]
              }
            }
          }
          frame True {
            n178 = One Button Dialog(message="Please abort currently running test if you wish to quit") -> ()  [unwired: 1 in, 1 out]
          }
        }
      }
      event Value Change {
        n179 = event-data() -> ()  [unwired: 1 in, 1 out]
        n180 = shared-variable ".\\Progress.lvlib\\Progress"() -> (w372:bool)  [unwired: 1 in, 1 out]
        n181 = case shown="True" w372 {
          tunnel: w374 -> [w378 w388]
          tunnel: [w379 w388] -> w373
          frame False {
            n182 = property on="Serial Number" class="Str"() -> ("Value"=w376:string)  [unwired: 2 in, 2 out]
            n183 = property on="User" class="Str"() -> ("Value"=w375:string)  [unwired: 2 in, 2 out]
            n184 = Bundle("Value"=w376, "Value"=w375) -> (w377:cluster{"Value":string, "Value":string})  [unwired: 1 in]
            n185 = Obtain Queue(name (unnamed)="OilMain", element data type=variant, error in (no error)=w378) -> (queue out=w383:refnum<queue>, error out=w384:errorcluster)  [unwired: 2 in, 1 out]
            n186 = call "State Machine - Enqueue State.vi"("error in (no error)"=w384, "Data"=w377, "State"="init test", "Queue In"=w383) -> ("error out"=w381:errorcluster, "Queue Out"=w380:refnum<queue>)  [unwired: 6 in]
            n187 = Release Queue(queue=w380, error in (no error)=w381) -> (error out=w379:errorcluster)  [unwired: 1 in, 2 out]
          }
          frame True {
            n188 = One Button Dialog(message="Test already in progress. Please wait until the test is over, or abort the test and start a new one.") -> ()  [unwired: 1 in, 1 out]
          }
        }
      }
      event Value Change {
        n189 = event-data() -> ()  [unwired: 1 in, 2 out]
        n190 = call "Get User Configuration File.vi"("error in (no error)"=w395) -> ("error out"=w394:errorcluster, "Config"=w390:T25)  [unwired: 9 in]
        n191 = Unbundle By Name(w390) -> ("Password"=w389:string)
        n192 = call "Get Password From User.vi"("error in"=w394, "password"=w389) -> ("error out"=w393:errorcluster, "Success?"=w392:bool)  [unwired: 8 in]
        n193 = case shown="True" w392 {
          tunnel: w393 -> [w396 w398]
          tunnel: [w396 w398] -> w391
          frame False {
            n194 = One Button Dialog(message="Invalid Password!" ("Message")) -> ()  [unwired: 1 in, 1 out]
          }
          frame True {
            n195 = call "Manual Mode.vi"() -> ()  [unwired: 12 in]
          }
        }
      }
      event Value Change {
        n196 = event-data() -> ()  [unwired: 1 in, 1 out]
        n197 = call "Read Configuration File.vi"("error in (no error)"=w402) -> ("error out"=w401:errorcluster, "User Config"=w400:T25)  [unwired: 9 in]
        n198 = Unbundle By Name(w400) -> ("Password"=w399:string)
        n199 = call "Get Password From User.vi"("error in"=w401, "password"=w399) -> ("error out"=w404:errorcluster, "Success?"=w403:bool)  [unwired: 8 in]
        n200 = case shown="True" w403 {
          tunnel: [w407 w411] -> w405
          tunnel: w404 -> [w407 w409]
          frame False {
            n201 = One Button Dialog(message="Invalid Password!" ("Message")) -> ()  [unwired: 1 in, 1 out]
          }
          frame True {
            n202 = call "Select Test Configuration.vi"("error in (no error)"=w409) -> ("error out"=w412:errorcluster, "Type"=w408:string, "Cancelled?"=w410:bool)  [unwired: 8 in]
            n203 = case shown="False" w410 {
              tunnel: w412 -> [w415 w422]
              tunnel: w408 -> [w414 _]
              tunnel: [w413 w422] -> w411
              frame False {
                n204 = case shown="\"Functionality\"" w414 {
                  tunnel: w415 -> [w417 w419 w421]
                  tunnel: [w416 w418 w420] -> w413
                  frame "Helium" {
                    n205 = call "Configure Helium Test.vi"("error in (no error)"=w417) -> ("error out"=w416:errorcluster)  [unwired: 10 in]
                  }
                  frame "Vacuum", Default {
                    n206 = call "Configure Vacuum Test.vi"("error in (no error)"=w419) -> ("error out"=w418:errorcluster)  [unwired: 10 in]
                  }
                  frame "Functionality" {
                    n207 = call "Configure Startup Test.vi"("error in (no error)"=w421) -> ("error out"=w420:errorcluster)  [unwired: 10 in]
                  }
                }
              }
              frame True {
              }
            }
          }
        }
      }
      event Value Change {
        n208 = event-data() -> ()  [unwired: 1 in, 1 out]
        n209 = shared-variable ".\\Progress.lvlib\\Progress"() -> (w423:bool)  [unwired: 1 in, 1 out]
        n210 = case shown="False" w423 {
          tunnel: w425 -> [w427 w431]
          tunnel: [w427 w430] -> w424
          frame False {
            n211 = One Button Dialog(message="No Test in Progress!") -> ()  [unwired: 1 in, 1 out]
          }
          frame True {
            n212 = Two Button Dialog(message="Are you sure you would like to abort the test?") -> (T button?=w429:bool)  [unwired: 2 in]
            n213 = case shown="True" w429 {
              tunnel: w431 -> [w432 w435]
              tunnel: [w432 w434] -> w430
              frame False {
              }
              frame True {
                n214 = shared-variable ".\\Abort.lvlib\\Abort"(TRUE ("Abort"), error in=w435) -> (error out=w434:errorcluster)
              }
            }
          }
        }
      }
    }
  }
  n215 = disable-structure shown="RUN_TIME_ENGINE==True" {
    disable-tunnel: w2 -> [_ _]
    frame condition #0 {
      n216 = Quit LabVIEW() -> ()  [unwired: 1 in]
    }
    frame condition #1 (active) {
    }
  }
  n217 = Release Queue(queue=w2, error in (no error)=w11) -> ()  [unwired: 1 in, 3 out]
